vi "ppanel_DO_stream_TTTR.vi"(4 "Correlation_settings":T2 {"Lag Settings"."time_start" items=["1 ps"=1, "10 ps"=10, "100 ps"=100, "1 ns"=1000, "10 ns"=10000, "100 ns"=100000, "1 us"=1000000, "10 us"=10000000, "100 us"=100000000, "1 ms"=1000000000, "10 ms"=10000000000, "100 ms"=100000000000, "1 s"=1000000000000, "10 s"=10000000000000, "100 s"=100000000000000]; "Lag Settings"."time_end" items=["1 ps"=1, "10 ps"=10, "100 ps"=100, "1 ns"=1000, "10 ns"=10000, "100 ns"=100000, "1 us"=1000000, "10 us"=10000000, "100 us"=100000000, "1 ms"=1000000000, "10 ms"=10000000000, "100 ms"=100000000000, "1 s"=1000000000000, "10 s"=10000000000000, "100 s"=100000000000000]}, 5 "Record Type":T1, 6 "stop_fifo_event":refnum<event-registration>, 7 "acq_time":i32, 8 "error in (no error)":errorcluster, 9 "action_for_records":T5, 10 "fifo_stream_path":path, 11 "hydraharp_panel in":refnum<class "picoharp_panel.lvclass">) -> (0 "error out":errorcluster, 3 "hydraharp_panel out":refnum<class "picoharp_panel.lvclass">)   [LabVIEW 2015, in "picoharp_panel.lvclass"]
uses:
  picoharp_panel.lvclass
  Hydraharp/hydraharp/hydraharp_action_on_records.ctl
  Hydraharp/hydraharp_panel/hpanel_correlation_settings.ctl
  Hydraharp/hydraharp/hydraharp_correlation_lag_settings.ctl
  Hydraharp/hydraharp/hydraharp_time_decades.ctl
  record_type.ctl
  picoharp/picoharp.lvclass
  Hydraharp/hydraharp_panel/hpanel_messages_to_panel_from_actor_loop.ctl
  picoharp/picoharp.lvclass/picoharp.ctl
  Picoquant_generic/processing_tasks_tdef.ctl
  Picoquant_generic/picoquant_generic.lvclass/picoquant_generic.ctl
  UI/panel_class/panel.lvclass
  Picoquant_generic/picoquant_generic.lvclass
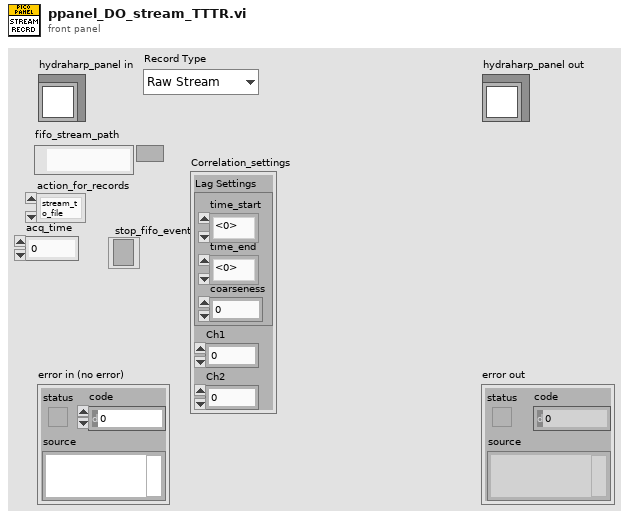
[diagram p1: front panel]
types:
  T1 = typedef "record_type.ctl" = enum16{"Raw Stream", "Processed Records (hdf5)"}
  T2 = typedef "hpanel_correlation_settings.ctl" = cluster{"Lag Settings":T3, "Ch1":u8, "Ch2":u8}
  T3 = typedef "hydraharp_correlation_lag_settings.ctl" = cluster{"time_start":T4, "time_end":T4, "coarseness":i64}
  T4 = typedef "hydraharp_time_decades.ctl" = i64
  T5 = typedef "hydraharp_action_on_records.ctl" = enum16{"stream_to_file", "correlate", "stream to file and correlate", "histogram"}
  T6 = typedef "hpanel_messages_to_panel_from_actor_loop.ctl" = enum16{"reenable_tasks"}
  T7 = typedef "processing_tasks_tdef.ctl" = enum16{"none", "correlate", "histogram"}
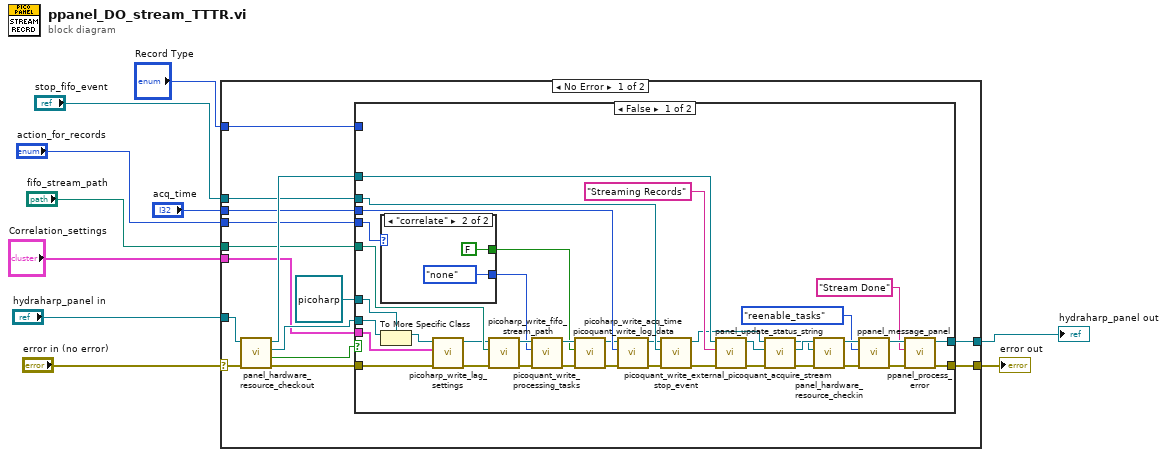
[diagram p0: block diagram]
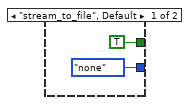
[diagram p2: hidden frame]
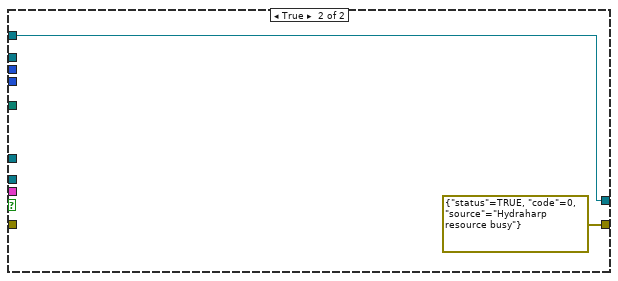
[diagram p3: hidden frame]
diagram:
  n1 = case shown="No Error" "error in (no error)" {
    selector: "error in (no error)" -> [w24 w71]
    tunnel: [w15 w71] -> w9
    tunnel: [w16 w70] -> w7
    tunnel: "hydraharp_panel in" -> [w25 w70]
    tunnel: "fifo_stream_path" -> [w18 _]
    tunnel: "action_for_records" -> [w17 _]
    tunnel: "acq_time" -> [w14 _]
    tunnel: "stop_fifo_event" -> [w13 _]
    tunnel: "Correlation_settings" -> [w12 _]
    tunnel: "Record Type" -> [w11 _]
    frame No Error {
      n2 = call "panel_hardware_resource_checkout.vi"("error in (no error)"=w24, "panel in"=w25) -> ("error out"=w20:errorcluster, "timed out?"=w21:bool, "hardware.lvclass"=w23:refnum<class "hardware.lvclass">, "panel out"=w19:refnum<class "picoharp_panel.lvclass">)  [unwired: 6 in]
      n3 = case shown="False" w21 {
        tunnel: w23 -> [w62 _]
        tunnel: refnum<class "picoharp.lvclass"> refnum ("picoharp.lvclass") -> [w63 _]
        tunnel: w20 -> [w54 _]
        tunnel: w19 -> [w60 w68]
        tunnel: w18 -> [w61 _]
        tunnel: w17 -> [w38 _]
        tunnel: [w46 w68] -> w16
        tunnel: [w45 errorcluster {"status"=TRUE, "code"=0, "source"="Hydraharp resource busy"} ("error out")] -> w15
        tunnel: w14 -> [w58 _]
        tunnel: w13 -> [w33 _]
        tunnel: w12 -> [w50 _]
        tunnel: w11 -> [_ _]
        frame False {
          n4 = case shown="\"correlate\"" w38 {
            tunnel: [TRUE FALSE] -> w37
            tunnel: [processing_tasks_tdef."none" ("processing tasks") processing_tasks_tdef."none" ("processing tasks")] -> w36
            frame "stream_to_file", Default {
            }
            frame "correlate" {
            }
          }
          n5 = To More Specific Class(target class=w63, reference=w62) -> (specific class reference=w52:refnum<class "picoharp.lvclass">)  [unwired: 1 in, 1 out]
          n6 = call "picoharp_write_lag_settings.vi"("error in (no error)"=w54, "lag_settings"=w50, "hydraharp in"=w52) -> ("error out"=w53:errorcluster, "hydraharp out"=w51:refnum<class "picoharp.lvclass">)  [unwired: 7 in]
          n7 = call "picoharp_write_fifo_stream_path.vi"("error in (no error)"=w53, "fifo_stream_path"=w61, "hydraharp in"=w51) -> ("error out"=w43:errorcluster, "hydraharp out"=w39:refnum<class "picoharp.lvclass">)  [unwired: 7 in]
          n8 = call "picoquant_write_processing_tasks.vi"("error in (no error)"=w43, "processing tasks"=w36, "picoquant_generic in"=w39) -> ("error out"=w44:errorcluster, "picoquant_generic out"=w40:refnum<class "picoharp.lvclass">)  [unwired: 7 in]
          n9 = call "picoquant_write_log_data.vi"("error in (no error)"=w44, "log data?"=w37, "picoquant_generic in"=w40) -> ("error out"=w42:errorcluster, "picoquant_generic out"=w41:refnum<class "picoharp.lvclass">)  [unwired: 7 in]
          n10 = call "picoharp_write_acq_time.vi"("error in (no error)"=w42, "acq_time"=w58, "hydraharp in"=w41) -> ("error out"=w35:errorcluster, "hydraharp out"=w32:refnum<class "picoharp.lvclass">)  [unwired: 7 in]
          n11 = call "picoquant_write_external_stop_event.vi"("error in (no error)"=w35, "external_stop_event"=w33, "picoquant_generic in"=w32) -> ("error out"=w34:errorcluster, "picoquant_generic out"=w28:refnum<class "picoharp.lvclass">)  [unwired: 7 in]
          n12 = call-dynamic "panel_update_status_string.vi"("error in (no error)"=w34, "String"="Streaming Records", "hydraharp_panel in"=w60) -> ("error out"=w27:errorcluster, "hydraharp_panel out"=w31:refnum<class "picoharp_panel.lvclass">)  [unwired: 7 in]
          n13 = call "picoquant_acquire_stream.vi"("error in (no error)"=w27, "picoquant_panel"=w31, "picoquant_generic in"=w28) -> ("error out"=w26:errorcluster, "panel out"=w30:refnum<class "picoharp_panel.lvclass">, "picoquant_generic out"=w29:refnum<class "picoharp.lvclass">)  [unwired: 6 in]
          n14 = call "panel_hardware_resource_checkin.vi"("error in (no error)"=w26, "hardware.lvclass"=w29, "panel in"=w30) -> ("error out"=w57:errorcluster, "panel out"=w56:refnum<class "picoharp_panel.lvclass">)  [unwired: 7 in]
          n15 = call "ppanel_message_panel.vi"("error in (no error)"=w57, "event data"=hpanel_messages_to_panel_from_actor_loop."reenable_tasks", "hydraharp_panel in"=w56) -> ("error out"=w49:errorcluster, "hydraharp_panel out"=w48:refnum<class "picoharp_panel.lvclass">)  [unwired: 7 in]
          n16 = call "ppanel_process_error.vi"("error in (no error)"=w49, "No Error Message"="Stream Done", "hydraharp_panel in"=w48) -> ("error out"=w45:errorcluster, "hydraharp_panel out"=w46:refnum<class "picoharp_panel.lvclass">)  [unwired: 7 in]
        }
        frame True {
        }
      }
    }
    frame Error {
    }
  }
  "error out" <- w9
  "hydraharp_panel out" <- w7
